vi "GUI_10TW_ESP.vi"() -> ()   [LabVIEW 2013]
uses:
  shared programs/GUI_Template/GUI_master/tcp_new_data_event.ctl
  shared programs/GUI_Template/GUI_master/tcp new data cluster.ctl
panel:
  in  "Status.Axis 3::1":T1(ring)=enum."Ready" caption="Status"
  in  "Home.Axis 3::1":dbl caption="Home" min=0.0 max=6.0 format="%_4f"
  in  "Power.Axis 3::1":enum16{"on", "off"}(ring)=enum."off" caption="Power"
  in  "Position.Axis 3::1":dbl caption="Position" min=0.0 max=2.9 format="%_4f"
  out "error IO 2":errorcluster
  out "tcp data event":T2
  in  "GUIdevice 1":string="10TW_ESP"
  in  "Status.Axis 2::1":T1(ring)=enum."Ready" caption="Status"
  in  "Status.Axis 1::1":T1(ring)=enum."Ready" caption="Status"
  in  "Home.Axis 2::1":dbl caption="Home" min=0.0 max=6.0 format="%_4f"
  in  "Power.Axis 2::1":enum16{"on", "off"}(ring)=enum."off" caption="Power"
  in  "Position.Axis 2::1":dbl caption="Position" min=0.0 max=2.9 format="%_4f"
  in  "Home.Axis 1::1":dbl caption="Home" min=0.0 max=6.0 format="%_4f"
  in  "Power.Axis 1::1":enum16{"on", "off"}(ring)=enum."off" caption="Power"
  in  "stop":bool
  in  "Position.Axis 1::1":dbl caption="Position" min=-5.0 max=2.9 format="%_4f"
  # "ESP301 GRAPHICAL USER INTERFACE"
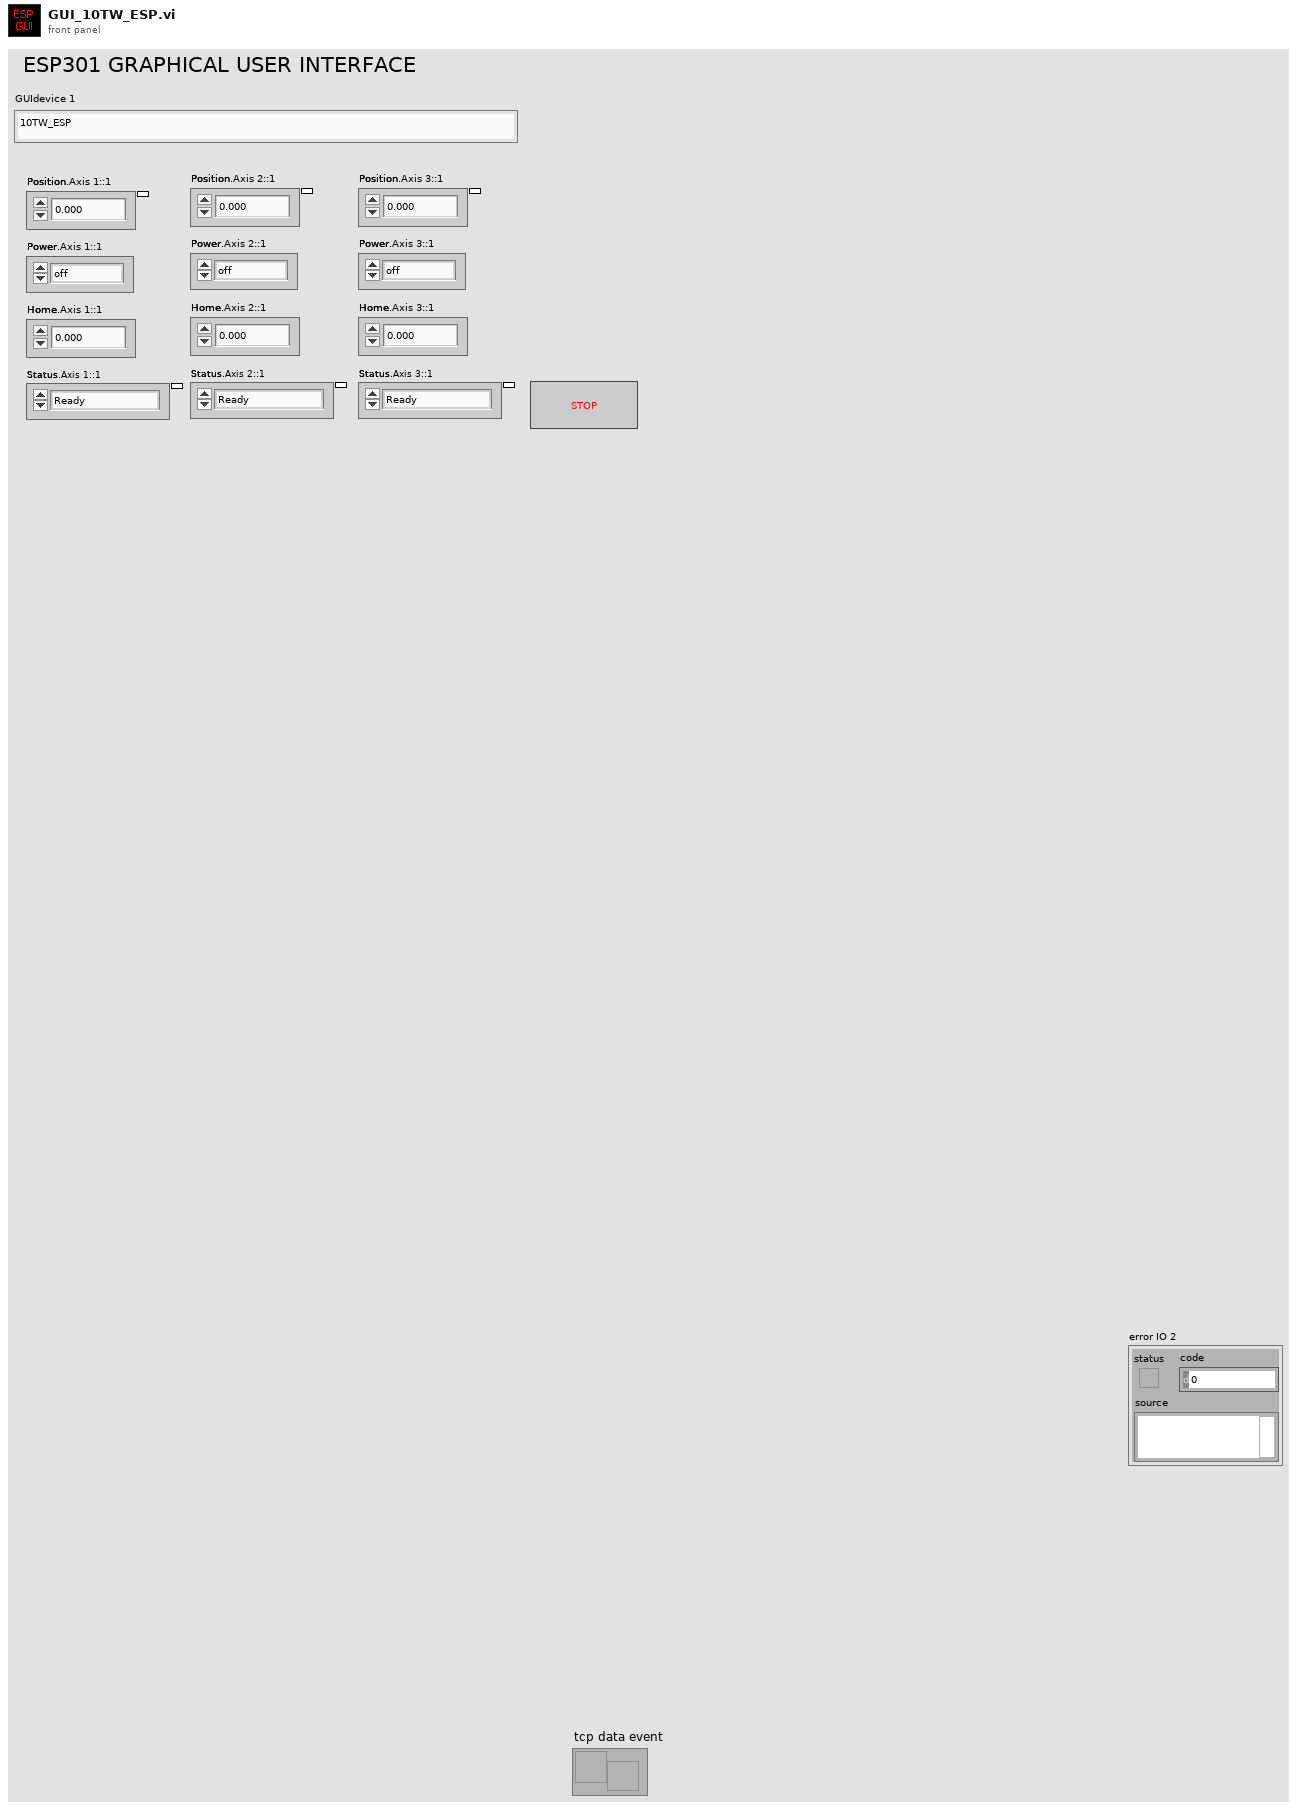
[diagram p1: front panel]
types:
  T1 = enum16{"Not referenced", "Homing", "Moving", "Ready"}
  T2 = typedef "tcp_new_data_event.ctl" = refnum<user-event>
  T3 = enum16{"Read", "Write", "ReadWrite", "BufferedRead", "BufferedReadWrite"}
  T4 = typedef "tcp new data cluster.ctl" = cluster{"EventEnum":enum16{"new data", "connection status update"}, "Device name":string}
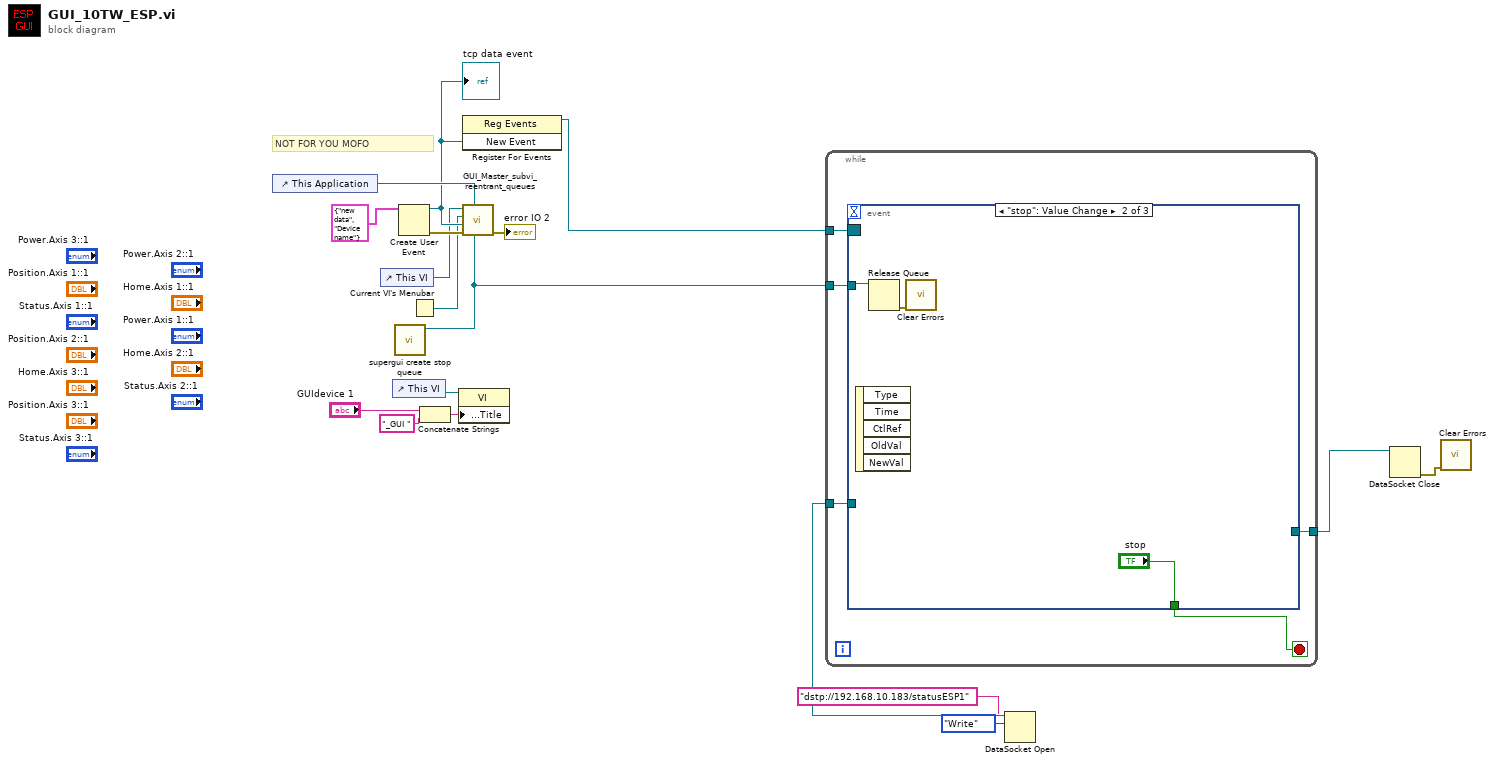
[diagram p0: block diagram]
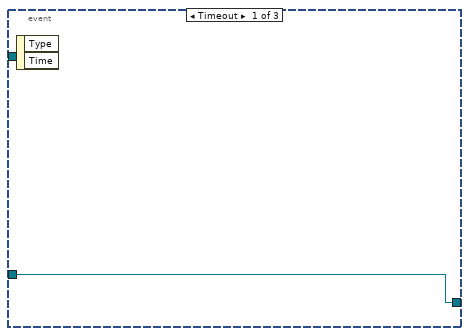
[diagram p2: hidden frame]
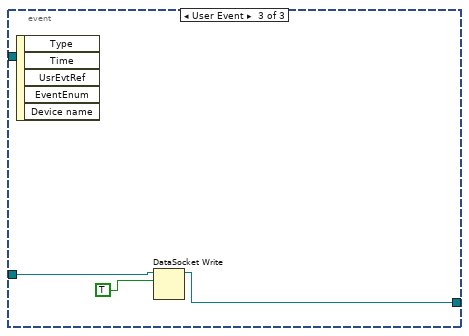
[diagram p3: hidden frame]
diagram:
  # "NOT FOR YOU MOFO"
  n1 = control-ref of="This Application"() -> (w18:refnum<vi>)
  n2 = control-ref of="This VI"() -> (w13:refnum<vi>)
  n3 = control-ref of="This VI"() -> (w4:refnum<vi>)
  n4 = call "supergui create stop queue.vi"() -> ("STOP Queue out"=w5:refnum<queue>)  [unwired: 11 in]
  n5 = Create User Event(user event datatype=T4 {"EventEnum"=enum."new data", "Device name"="Device name"} ("New Event")) -> (user event=w17:refnum<user-event>, error out=w16:errorcluster)  [unwired: 1 in]
  "tcp data event" <- w17
  n6 = Current VI's Menubar() -> (w14:refnum<k9>)
  n7 = Concatenate Strings("GUIdevice 1", "_GUI ") -> (w3:string)
  n8 = property class="VI"(reference=w4, "Front Panel.Title"=w3) -> ()  [unwired: 1 in, 2 out]
  n9 = register-events(w17) -> (reference out=w11:refnum<event-registration>)  [unwired: 2 in, 1 out]
  n10 = call "GUI_Master_subvi_reentrant_queues.vi"("STOP Queue in"=w5, "This Application"=w18, "error in (no error)"=w16, "tcp data event"=w17, "Caller menu reference"=w14, "Caller VI ref"=w13) -> ("error out"=→"error IO 2":errorcluster)  [unwired: 5 in]
  n11 = DataSocket Open(10:T3."Write" ("mode"), 11:"dstp://192.168.10.183/statusESP1") -> (3:w10:refnum<k13>)  [unwired: 2 in, 1 out]
  n12 = while {
    tunnel: w11 -> [w23]
    tunnel: w10 -> [w22]
    tunnel: [w21] -> w7
    tunnel: w5 -> [w19]
    stop <- w20 stop-if-true
    n13 = event shown="[1] \"stop\": Value Change" {
      selector: w23 -> [_ _ _]
      dyn-events: _ -> [_ _ _]
      timeout: _ -> [_ _ _]
      tunnel: w22 -> [w24 _ w30]
      tunnel: [w24 _ w29] -> w21
      tunnel: [_ "stop" _] -> w20
      tunnel: w19 -> [_ w26 _]
      event Timeout {
        n14 = event-data() -> ()  [unwired: 1 in, 2 out]
      }
      event "stop": Value Change {
        n15 = event-data() -> ()  [unwired: 1 in, 5 out]
        n16 = Release Queue(queue=w26) -> (error out=w25:errorcluster)  [unwired: 2 in, 2 out]
        n17 = call <vilib>:"Clear Errors.vi"("error in (no error)"=w25) -> ()  [unwired: 6 in, 1 out]
      }
      event User Event {
        n18 = event-data() -> ()  [unwired: 1 in, 5 out]
        n19 = DataSocket Write(10:TRUE ("status"), 11:w30) -> (3:w29:refnum<k13>)  [unwired: 2 in, 2 out]
      }
    }
  }
  n20 = DataSocket Close(11:w7) -> (0:w6:errorcluster)  [unwired: 2 in, 1 out]
  n21 = call <vilib>:"Clear Errors.vi"("error in (no error)"=w6) -> ()  [unwired: 6 in, 1 out]
